vi "Shortest Distance Absolute.vi"(10 "Target":dbl(knob) scale=0.0..360.0, 11 "Current":dbl(knob) scale=0.0..360.0) -> (3 "Angle to Rotate":dbl)   [LabVIEW 2014]
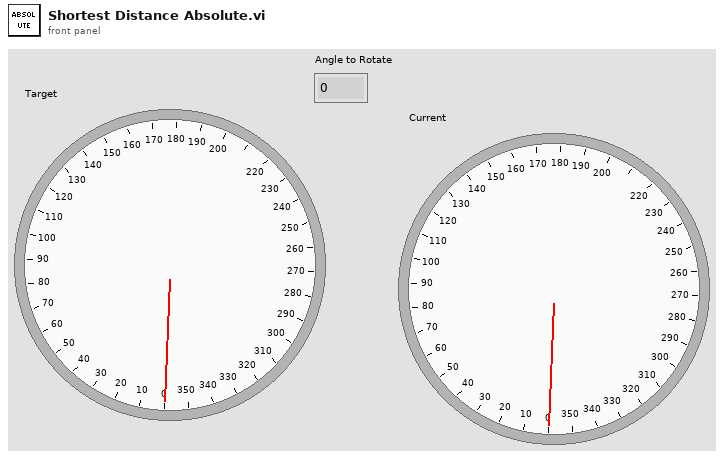
[diagram p1: front panel]
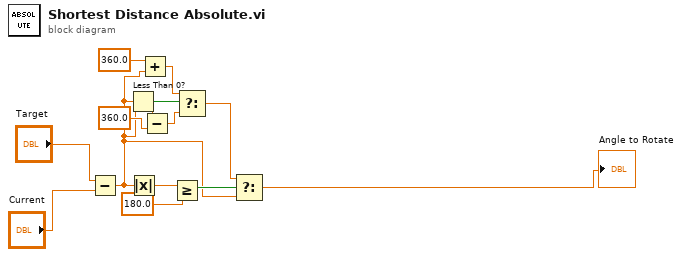
[diagram p0: block diagram]
diagram:
  n1 = Subtract(x="Target", y="Current") -> (x-y=w1:dbl)
  n2 = Less Than 0?(x=w1) -> (x < 0?=w6:bool)
  n3 = Absolute Value(x=w1) -> (abs(x)=w11:dbl)
  n4 = Add(x=360.0, y=w1) -> (x+y=w4:dbl)
  n5 = Subtract(x=w1, y=360.0 ("x")) -> (x-y=w5:dbl)
  n6 = Greater Or Equal?(x=w11, y=180.0) -> (x >= y?=w9:bool)
  n7 = Select(t=w4, s=w6, f=w5) -> (s? t:f=w7:dbl)
  n8 = Select(t=w7, s=w9, f=w1) -> (s? t:f=→"Angle to Rotate":dbl)
